vi "INI_RFID.vi"(3 "MCListbox Ref":refnum<vi>, 8 "MListBox Row":u16=2 max=8, 10 "Device INI Config File Path":path=path "D:/LABVIEW/SEQUENSER_SNA/Ver_12/INI/DeviceConfig.ini") -> (0 "error out":errorcluster, 1 "ComPort":refnum<visa-resource-name>, 2 "Dev OK":bool)   [LabVIEW 2018]
uses:
  <vilib>/Utility/miscctls.llb/LVRowAndColumnTypeDef.ctl
  <vilib>/Utility/config.llb/Read Key (String).vi
  <vilib>/Utility/config.llb/NI_LVConfig.lvlib
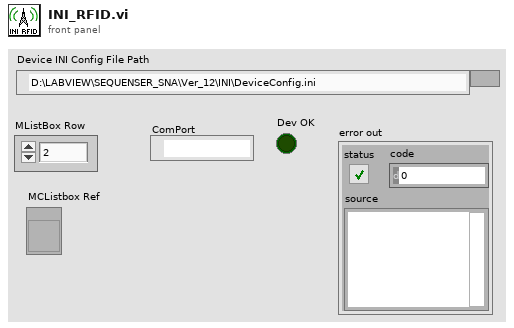
[diagram p1: front panel]
types:
  T1 = typedef "LVRowAndColumnTypeDef.ctl" = cluster{"Row":i32, "Column":i32}
  T2 = typedef "NI_LVConfig.lvlib/Config Data RefNum.ctl" = refnum<k1>
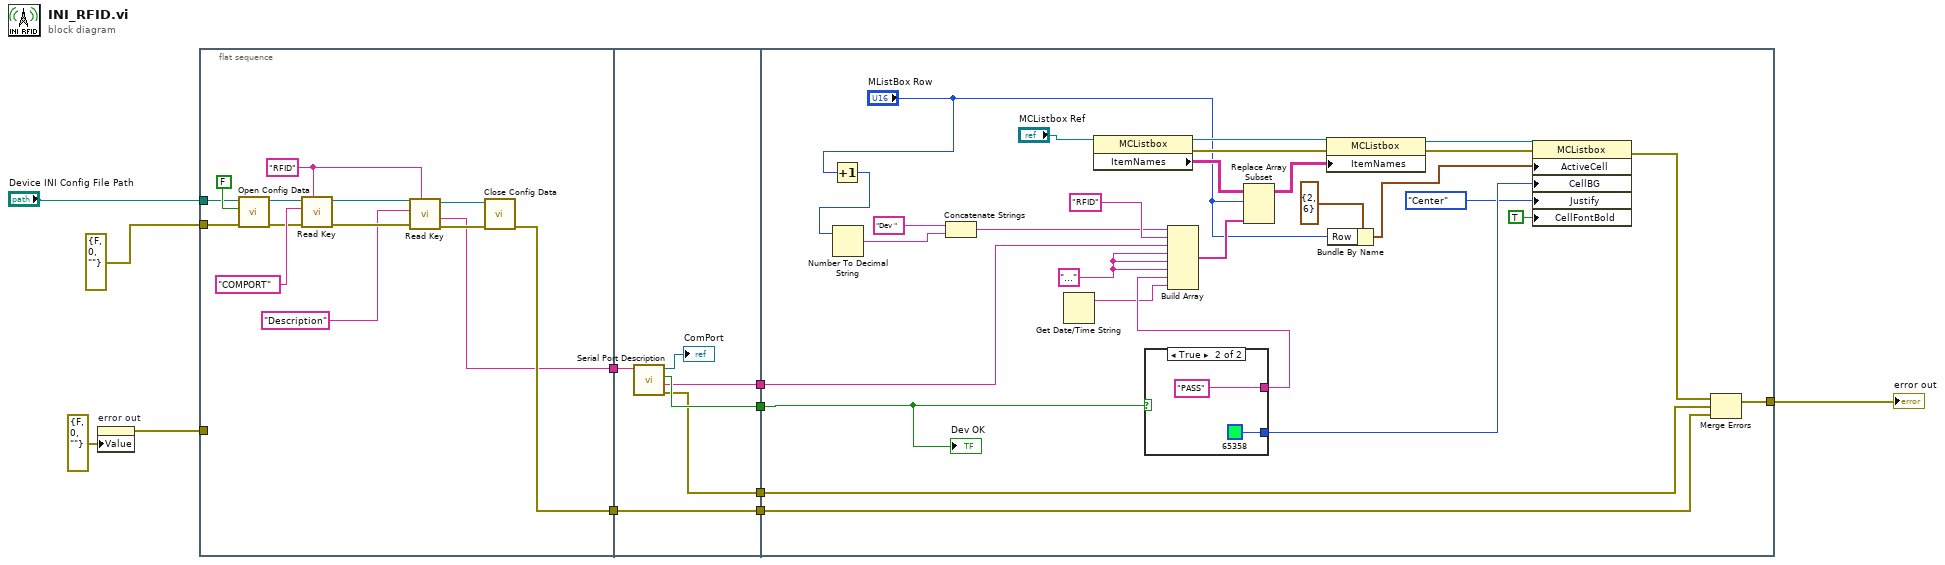
[diagram p0: block diagram]
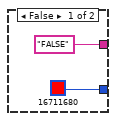
[diagram p2: hidden frame]
diagram:
  n1 = property on="error out" class="Clust (strict)"("Value"=errorcluster {"status"=FALSE, "code"=0, "source"=""} ("error out")) -> (error out=w9:errorcluster)  [unwired: 2 in, 1 out]
  n2 = flat-sequence {
    tunnel: "Device INI Config File Path" -> [w21]
    tunnel: [w20] -> w11
    tunnel: w9 -> [_]
    tunnel: errorcluster {"status"=FALSE, "code"=0, "source"=""} ("error constant") -> [w19]
    tunnel: [w13] -> w5
    tunnel: w11 -> [w28]
    tunnel: w5 -> [w27]
    tunnel: [w31] -> w4
    tunnel: [w30] -> w3
    tunnel: [w28] -> w2
    tunnel: [w26] -> w1
    tunnel: [w35] -> w7
    tunnel: w4 -> [w38]
    tunnel: w3 -> [w36]
    tunnel: w2 -> [w32]
    tunnel: w1 -> [w33]
    frame #0 {
      w14 = "RFID" ("section")
      n3 = call <vilib>:"Open Config Data.vi"("error in (no error)"=w19, "create file if necessary (T)"=FALSE, "configuration file path"=w21) -> ("error out"=w24:errorcluster, "refnum"=w23:T2)  [unwired: 6 in, 1 out]
      n4 = call-poly <vilib>:"Read Key.vi"("section"=w14, "error in (no error)"=w24, "key"="COMPORT", "refnum"=w23) -> ("error out"=w16:errorcluster, "refnum out"=w18:T2)  [unwired: 4 in, 2 out]
      n5 = call-poly <vilib>:"Read Key.vi"("section"=w14, "error in (no error)"=w16, "key"="Description", "refnum"=w18) -> ("error out"=w15:errorcluster, "value"=w13:string, "refnum out"=w17:T2)  [unwired: 4 in, 1 out]
      n6 = call <vilib>:"Close Config Data.vi"("error in (no error)"=w15, "refnum"=w17) -> ("error out"=w20:errorcluster)  [unwired: 8 in, 1 out]
    }
    frame #1 {
      n7 = call "Serial Port Description.vi"("Dev Description"=w27) -> ("error out"=w26:errorcluster, "Device"=w30:string, "OK?"=w31:bool, "VISA resource name"=→"ComPort":refnum<visa-resource-name>)  [unwired: 7 in]
    }
    frame #2 {
      w37 = "..."
      n8 = Increment(x="MListBox Row") -> (x+1=w40:u16)
      n9 = Number To Decimal String(number=w40) -> (decimal integer string=w57:string)  [unwired: 1 in]
      n10 = Concatenate Strings("Dev ", w57) -> (w58:string)
      n11 = Get Date/Time String() -> (date string=w50:string)  [unwired: 3 in, 1 out]
      n12 = property class="MCListbox"(reference="MCListbox Ref") -> (reference out=w48:refnum<vi>, error out=w47:errorcluster, "ItemNames"=w46:string[][])  [unwired: 1 in]
      n13 = case shown="True" w38 {
        tunnel: [u32 16711680 u32 65358] -> w53
        tunnel: ["FALSE" ("element") "PASS" ("element")] -> w54
        frame False {
        }
        frame True {
        }
      }
      n14 = Build Array(w58, "RFID", w36, w37, w37, w37, w54, w50) -> (w44:string[])
      n15 = Replace Array Subset(array=w46, new element=w44, index (row)="MListBox Row") -> (w45:string[][])  [unwired: 1 in]
      n16 = property class="MCListbox"(reference=w48, error in=w47, "ItemNames"=w45) -> (reference out=w43:refnum<vi>, error out=w42:errorcluster)
      n17 = Bundle By Name(cluster=T1 {"Row"=2, "Column"=6} ("Active Cell:Active Cell"), "Row"="MListBox Row") -> (w52:T1)
      n18 = property class="MCListbox"(reference=w43, error in=w42, "ActiveCell"=w52, "CellBG"=w53, "Justify"=enum16{"Left", "Center", "Right"}."Center" ("Active Cell:Cell Justification"), "CellFontBold"=TRUE ("Active Cell:Cell Font:Bold")) -> (error out=w34:errorcluster)  [unwired: 1 out]
      n19 = Merge Errors(w34, w33, w32) -> (w35:errorcluster)
      "Dev OK" <- w38
    }
  }
  "error out" <- w7
